vi "4-4.vi"(0 "数值":i32, 1 "use system alert? (T)":bool=TRUE caption="使用系统警报？(T)", 2 "duration (msec)":u32 caption="持续时间（毫秒）", 3 "frequency (Hz)":u32 caption="频率(Hz)") -> ()   [LabVIEW 2017]
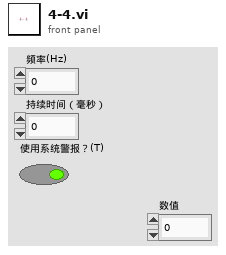
[diagram p1: front panel]
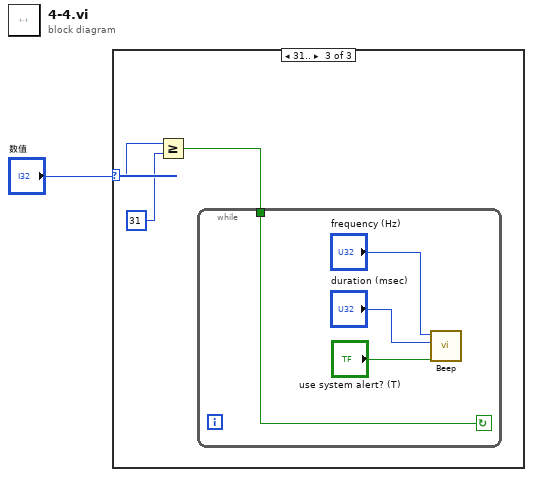
[diagram p0: block diagram]
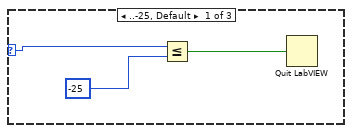
[diagram p2: hidden frame]
diagram:
  n1 = case shown="31.." "数值" {
    selector: "数值" -> [w3 _ w7]
    frame ..-25, Default {
      n2 = Less Or Equal?(x=w3, y=-25) -> (x <= y?=w4:bool)
      n3 = Quit LabVIEW(quit? (T)=w4) -> ()
    }
    frame -24..30 {
    }
    frame 31.. {
      n4 = Greater Or Equal?(x=w7, y=31) -> (x >= y?=w5:bool)
      n5 = while {
        tunnel: w5 -> [w8]
        stop <- w8 continue-if-true
        n6 = call <vilib>:"Beep.vi"("use system alert? (T)"="use system alert? (T)", "duration (msec)"="duration (msec)", "frequency (Hz)"="frequency (Hz)") -> ()  [unwired: 9 in]
      }
    }
  }
